vi "lab2_new.vi"() -> ()   [LabVIEW 2021]
panel:
  out "N!":u64
  in  "N":u64
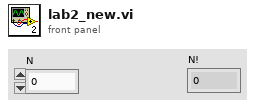
[diagram p1: front panel]
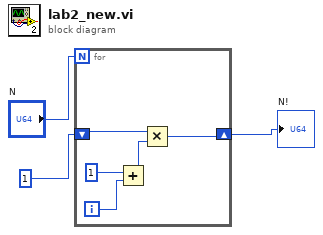
[diagram p0: block diagram]
diagram:
  n1 = for {
    N: "N" -> [_]
    shift-right: [w6] -> w3
    shift-left: 1 -> [w7]
    i -> [w5]
    n2 = Add(x=1, y=w5) -> (x+y=w8:i32)
    n3 = Multiply(x=w7, y=w8) -> (x*y=w6:i32)
  }
  "N!" <- w3
